vi "Build Spec-Type.vi"(8 "error in (no error)":errorcluster, 10 "Type":string="Packed Library", 11 "Path to project":path) -> (0 "error out":errorcluster)   [LabVIEW 2021]
uses:
  <vilib>/AppBuilder/AB_API_Simple/Build (path).vi
  <vilib>/AppBuilder/AB_API_Simple/NI_App_Builder_API.lvlib
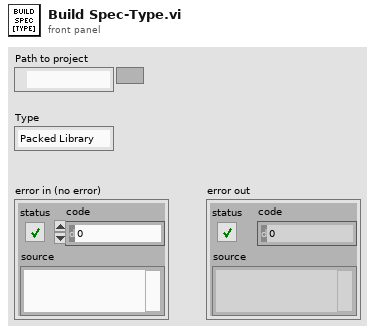
[diagram p1: front panel]
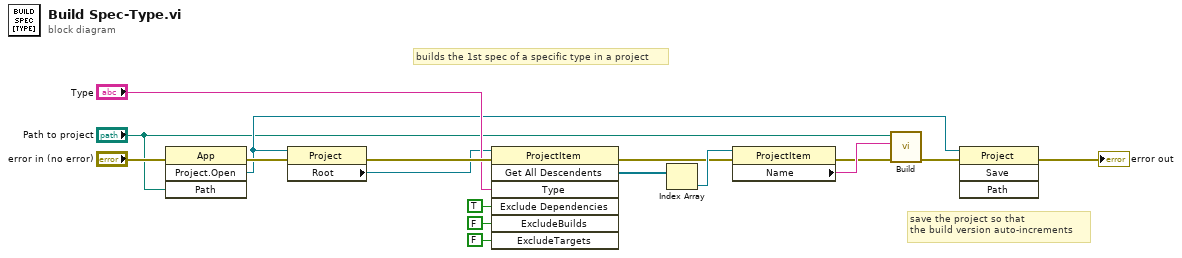
[diagram p0: block diagram]
diagram:
  # "save the project so that\nthe build version auto-increments"
  # "builds the 1st spec of a specific type in a project"
  n1 = invoke class="App" method="Project.Open"(error in="error in (no error)", "Path"="Path to project") -> (error out=w5:errorcluster, "Project:Open"=w3:refnum<vi>)  [unwired: 2 in, 2 out]
  n2 = property class="Project"(reference=w3, error in=w5) -> (error out=w11:errorcluster, "Root"=w6:refnum<vi>)  [unwired: 1 out]
  n3 = invoke class="ProjectItem" method="Get All Descendents"(reference=w6, error in=w11, "Type"="Type", "Exclude Dependencies"=TRUE ("ExcludeDependencies"), "ExcludeBuilds"=FALSE, "ExcludeTargets"=FALSE) -> (error out=w12:errorcluster, "All Descendents"=w13:refnum<vi>[])  [unwired: 1 in, 5 out]
  n4 = Index Array(array=w13) -> (element=w14:refnum<vi>)  [unwired: 1 in]
  n5 = property class="ProjectItem"(reference=w14, error in=w12) -> (error out=w15:errorcluster, "Name"=w16:string)  [unwired: 1 out]
  n6 = call-poly <vilib>:"Build.vi"("error in (no error)"=w15, "Name of build specification (if empty: build all)"=w16, "Path to project"="Path to project") -> ("error out"=w4:errorcluster)  [unwired: 7 in, 1 out]
  n7 = invoke class="Project" method="Save"(reference=w3, error in=w4) -> (error out=→"error out":errorcluster)  [unwired: 2 in, 3 out]
